vi "DataUnit2.vi"(11 "DataName":string) -> (2 "Unit":string, 3 "DataName(dup)":string)   [LabVIEW 2020, in "CSM-TagDashboard.lvlib"]
uses:
  CSM-TagDashboard.lvlib
  <userlib>/_NEVSTOP/Communicable State Machine(CSM)/addons/INI-Static-Variable-Support/INI-Static-Variable-Support.lvlib
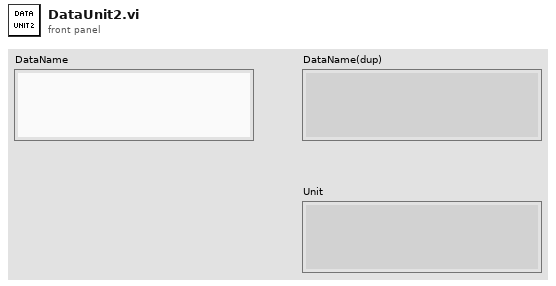
[diagram p1: front panel]
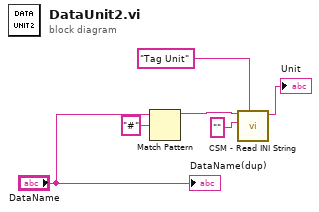
[diagram p0: block diagram]
diagram:
  n1 = Match Pattern(string="DataName", regular expression="#") -> (before substring=w2:string)  [unwired: 1 in, 3 out]
  n2 = call <userlib>:"CSM - Read INI String.vi"("Section Name (\"\" as Default)"="Tag Unit" ("Section Name(\"\" as Default)"), "Default Value"="" ("y"), "Variable Name"=w2) -> ("Value"=→"Unit":string)  [unwired: 4 in, 2 out]
  "DataName(dup)" <- "DataName"
